vi "Global_SM_Data Out.vi"() -> ()   [LabVIEW 2017, in "Overlords.lvlib"]
uses:
  Overlords.lvlib
  Cluster_SM Status.ctl
  ENUM_Overloard State.ctl
  ENUM _Overloard Shooter States.ctl
  ENUM_Overloard Gear States.ctl
  ENUM_Overloard Climb States.ctl
panel:
  in  "SM_Status":T1={"Task Complete"=FALSE, "Current Overlord State"=enum."Idle", "Wanted State"=enum."Idle", "Overloard Shooter States"=enum."Complete", "Overlord Gear State"=enum."Complete", "Overlord Climber State"=enum."Complete"}
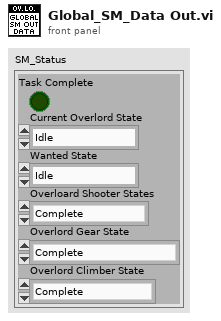
[diagram p1: front panel]
types:
  T1 = typedef "Overlords.lvlib/Cluster_SM Status.ctl" = cluster{"Task Complete":bool, "Current Overlord State":T2, "Wanted State":T2, "Overloard Shooter States":T3, "Overlord Gear State":T4, "Overlord Climber State":T5}
  T2 = typedef "Overlords.lvlib/ENUM_Overloard State.ctl" = enum16{"Idle", "High Shot", "Low Shot", "Place Gear", "Climb"}
  T3 = typedef "Overlords.lvlib/ENUM _Overloard Shooter States.ctl" = enum16{"Startup", "Idle", "Locate Target", "Wait To Be in Position", "Shooting", "Complete"}
  T4 = typedef "Overlords.lvlib/ENUM_Overloard Gear States.ctl" = enum16{"Startup", "Idle", "Detect Target", "Verticle Track (Sonar)", "Encoder Setup", "Verticle Track (Encoder)", "Gear Present", "Gear Present Counter", "Verticle Backword Track", "Complete"}
  T5 = typedef "Overlords.lvlib/ENUM_Overloard Climb States.ctl" = enum16{"Startup", "Idle", "Check Time", "Check Statis", "Complete"}
diagram:
